vi "Set Temporary String Property.vi"(8 "error in (no error)":errorcluster, 9 "value":string, 10 "property name":string, 11 "Item Ref in":T1 format="%.0x") -> (0 "error out":errorcluster, 3 "Item Ref out":T1 format="%.0x")   [LabVIEW 2020, in "Routing and Faulting System Explorer.lvlib"]
uses:
  Routing and Faulting System Explorer.lvlib
  <vilib>/NI VeriStand/Custom Device API/Custom Device Item Ref.ctl
  NationalInstruments.VeriStand.SystemStorage
  Scripting/Routing and Faulting Scripting.lvlib
  <vilib>/NI VeriStand/Custom Device API/Custom Device API.lvlib
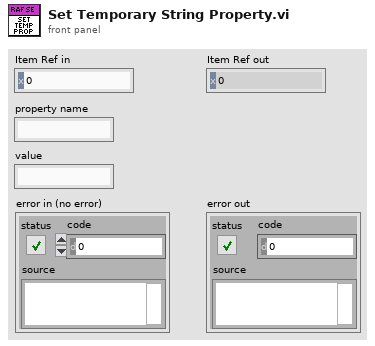
[diagram p1: front panel]
types:
  T1 = typedef "Custom Device API.lvlib/Custom Device Item Ref.ctl" = u64
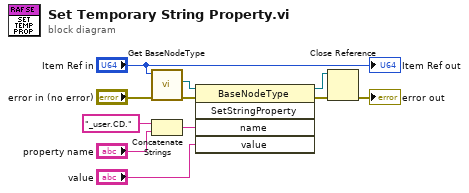
[diagram p0: block diagram]
diagram:
  n1 = call "Get BaseNodeType.vi"("error in"="error in (no error)", "item in"="Item Ref in") -> ("error out"=w2:errorcluster, "BaseNodeType"=w9:refnum<k24>)  [unwired: 7 in, 1 out]
  n2 = Concatenate Strings("_user.CD." ("string"), "property name") -> (w8:string)
  n3 = invoke class="BaseNodeType" method="SetStringProperty"(reference=w9, error in=w2, "name"=w8, "value"="value") -> (reference out=w4:refnum<k24>, error out=w5:errorcluster)  [unwired: 1 in, 3 out]
  n4 = Close Reference(reference=w4, error in (no error)=w5) -> (error out=→"error out":errorcluster)
  "Item Ref out" <- "Item Ref in"
